vi "niRFUtil LCAPI Copy 1D Array (1 I32, 6 DBL).vi"(0 "Source0 1D Array (I32)":i32[](array[numeric]), 1 "Source1 1D Array (DBL)":dbl[](array[numeric]) format="%.2f", 2 "Source2 1D Array (DBL)":dbl[](array[numeric]) format="%.2f", 3 "Source3 1D Array (DBL)":dbl[](array[numeric]) format="%.2f", 4 "Source4 1D Array (DBL)":dbl[](array[numeric]) format="%.2f", 5 "error in (no error)":errorcluster, 6 "Source5 1D Array (DBL)":dbl[](array[numeric]) format="%.2f", 7 "Data Copy Descriptor":u64, 8 "Source6 1D Array (DBL)":dbl[](array[numeric]) format="%.2f") -> (10 "Source6 Out":dbl[](array[numeric]) format="%.2f", 12 "Source5 Out":dbl[](array[numeric]) format="%.2f", 14 "Source0 Out":i32[](array[numeric]), 15 "Source1 Out":dbl[](array[numeric]) format="%.2f", 16 "Source2 Out":dbl[](array[numeric]) format="%.2f", 17 "Source3 Out":dbl[](array[numeric]) format="%.2f", 18 "Source4 Out":dbl[](array[numeric]) format="%.2f", 19 "error out":errorcluster)   [LabVIEW 2015, in "niRFUtil.lvlib"]
uses:
  niRFUtil.lvlib
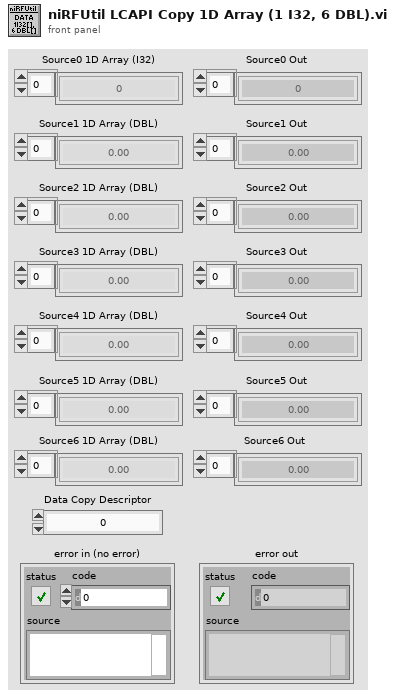
[diagram p1: front panel]
types:
  T1 = cluster{"status":bool, "return type":i32, "errorString":string}
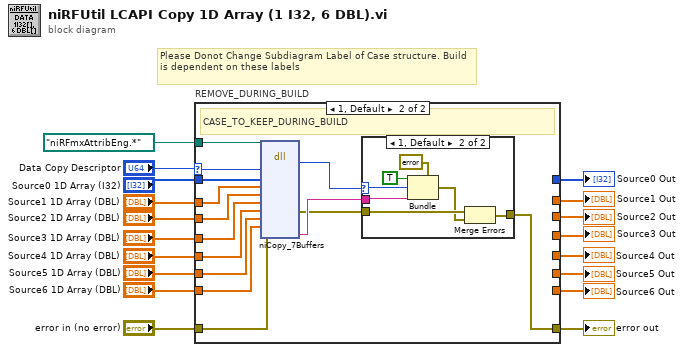
[diagram p0: block diagram]
diagram:
  # "Please Donot Change Subdiagram Label of Case structure. Build is dependent on these labels"
  n1 = case "REMOVE_DURING_BUILD" shown="1, Default" "Data Copy Descriptor" {
    selector: "Data Copy Descriptor" -> [_ w30]
    tunnel: "error in (no error)" -> [w21 w39]
    tunnel: "Source1 1D Array (DBL)" -> [w25 w38]
    tunnel: "Source2 1D Array (DBL)" -> [w24 w37]
    tunnel: "Source3 1D Array (DBL)" -> [w23 w36]
    tunnel: "Source4 1D Array (DBL)" -> [w22 w35]
    tunnel: "Source0 1D Array (I32)" -> [w26 w34]
    tunnel: [w26 _] -> w9
    tunnel: [w25 _] -> w11
    tunnel: [w24 _] -> w8
    tunnel: [w23 _] -> w10
    tunnel: [w22 _] -> w7
    tunnel: [w21 w40] -> w6
    tunnel: path "niRFmxAttribEng.*" ("path in") -> [_ w29]
    tunnel: "Source5 1D Array (DBL)" -> [w20 w28]
    tunnel: "Source6 1D Array (DBL)" -> [w19 w27]
    tunnel: [w20 _] -> w2
    tunnel: [w19 _] -> w1
    frame 0 {
      # "Development"
    }
    frame 1, Default {
      # "CASE_TO_KEEP_DURING_BUILD"
      n2 = dll-call lib="niRFmxAttribEng.*" fn="niCopy_7Buffers"(path in=w29, error in=w39, "dataCopyDescriptor"=w30, "source0"=w34, "source1"=w38, "source2"=w37, "source3"=w36, "source4"=w35, "source5"=w28, "source6"=w27) -> (error out=w31:errorcluster, "return type"=w33:i32, "errorString"=w32:string)  [unwired: 10 in, 1 out]
      n3 = case shown="1, Default" w33 {
        selector: w33 -> [_ w47]
        tunnel: w32 -> [_ w46]
        tunnel: w31 -> [w41 w44]
        tunnel: [w41 w45] -> w40
        frame 0 {
        }
        frame 1, Default {
          n4 = Bundle(cluster=T1 {"status"=FALSE, "return type"=0, "errorString"=""}, "status"=TRUE, "return type"=w47, "errorString"=w46) -> (w43:T1)
          n5 = Merge Errors(w44, w43) -> (w45:errorcluster)
        }
      }
    }
  }
  "error out" <- w6
  "Source0 Out" <- w9
  "Source1 Out" <- w11
  "Source2 Out" <- w8
  "Source3 Out" <- w10
  "Source4 Out" <- w7
  "Source5 Out" <- w2
  "Source6 Out" <- w1
